vi "MSScript_SubVI_IsARegularVarArray.vi"(9 "VarString in":string) -> (1 "Variable simbol no found":bool, 2 "irregular":bool, 3 "VarString out":string)   [LabVIEW 2018, in "MSScript.lvclass"]
uses:
  MSScript.lvclass
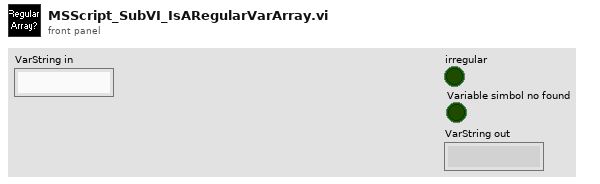
[diagram p1: front panel]
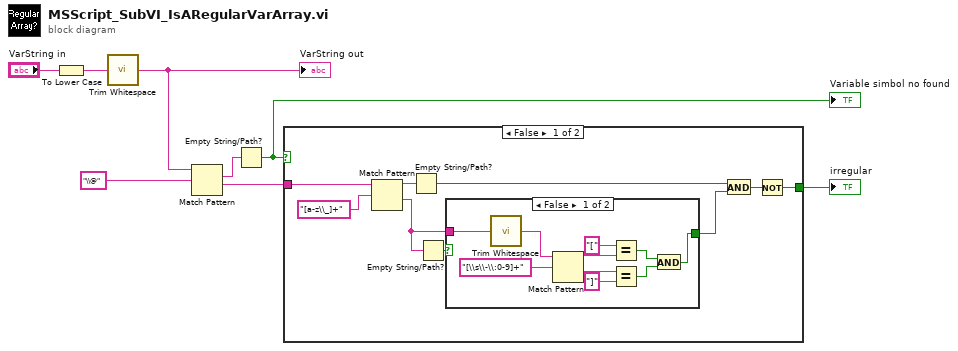
[diagram p0: block diagram]
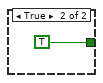
[diagram p3: hidden frame]
diagram:
  n1 = To Lower Case(string="VarString in") -> (all lower case string=w2:string)
  n2 = call <vilib>:"Trim Whitespace.vi"("string"=w2) -> ("trimmed string"=w1:string)  [unwired: 1 in]
  "VarString out" <- w1
  n3 = Match Pattern(string=w1, regular expression="\\@") -> (match substring=w7:string, after substring=w6:string)  [unwired: 1 in, 2 out]
  n4 = Empty String/Path?(string/path=w7) -> (empty?=w3:bool)
  "Variable simbol no found" <- w3
  n5 = case shown="False" w3 {
    tunnel: [w13 TRUE] -> w4
    tunnel: w6 -> [w12 _]
    frame False {
      n6 = Match Pattern(string=w12, regular expression="[a-z\\_]+") -> (before substring=w16:string, after substring=w9:string)  [unwired: 1 in, 2 out]
      n7 = Empty String/Path?(string/path=w16) -> (empty?=w15:bool)
      n8 = Empty String/Path?(string/path=w9) -> (empty?=w11:bool)
      n9 = case shown="False" w11 {
        selector: w11 -> [_ w28]
        tunnel: [w18 w28] -> w10
        tunnel: w9 -> [w24 _]
        frame False {
          n10 = call <vilib>:"Trim Whitespace.vi"("string"=w24) -> ("trimmed string"=w23:string)  [unwired: 1 in]
          n11 = Match Pattern(string=w23, regular expression="[\\s\\-\\:0-9]+") -> (before substring=w26:string, after substring=w25:string)  [unwired: 1 in, 2 out]
          n12 = Equal?(x="[", y=w26) -> (x = y?=w20:bool)
          n13 = Equal?(x=w25, y="]") -> (x = y?=w19:bool)
          n14 = And(x=w20, y=w19) -> (x .and. y?=w18:bool)
        }
        frame True {
        }
      }
      n15 = And(x=w15, y=w10) -> (x .and. y?=w14:bool)
      n16 = Not(x=w14) -> (.not. x?=w13:bool)
    }
    frame True {
    }
  }
  "irregular" <- w4
